vi "ByteArrayToHexStringArray.vi"(5 "ByteArrayIn":u8[](array[numeric]) format="%02x") -> (2 "HexStringArrayOut":string)   [LabVIEW 2011, in "GenericCanAdapterClass.lvclass"]
uses:
  GenericCanAdapterClass.lvclass
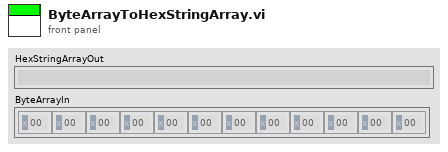
[diagram p1: front panel]
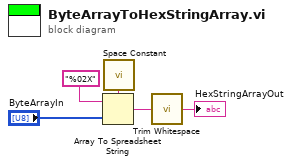
[diagram p0: block diagram]
diagram:
  n1 = call <vilib>:"Space Constant.vi"() -> ("String"=w4:string)
  n2 = Array To Spreadsheet String(delimiter (Tab)=w4, array="ByteArrayIn", 3:"%02X" ("format string")) -> (spreadsheet string=w3:string)
  n3 = call <vilib>:"Trim Whitespace.vi"("string"=w3) -> ("trimmed string"=→"HexStringArrayOut":string)  [unwired: 1 in]
